vi "transferScanPatternToTarget.vi"(8 "error in (no error)":errorcluster, 10 "FPGA VI ref":T1, 11 "Queues":T2) -> (0 "error out":errorcluster)   [LabVIEW 2010]
uses:
  internal_queues.ctl
  line_info.ctl
  volume_with_lines.ctl
  volume_info.ctl
  kalman_result_scaled.ctl
  projection buffers.ctl
  location3D.ctl
  spot location.ctl
  FPGA_ref.ctl
  <vilib>/rvi/interface/nirviMethod/nirviMethod.xnode
  <vilib>/rvi/interface/common/niFpgaNodeNameForErrorReporting.ctl
  <vilib>/rvi/errors/niLvFpgaWhatHappensToTopLevelVI.ctl
  <vilib>/Utility/error.llb/Error Cluster From Error Code.vi
  <vilib>/rvi/errors/niLvFpgaAdjustHostInterfaceError.vi
  NiFpgaLv.dll
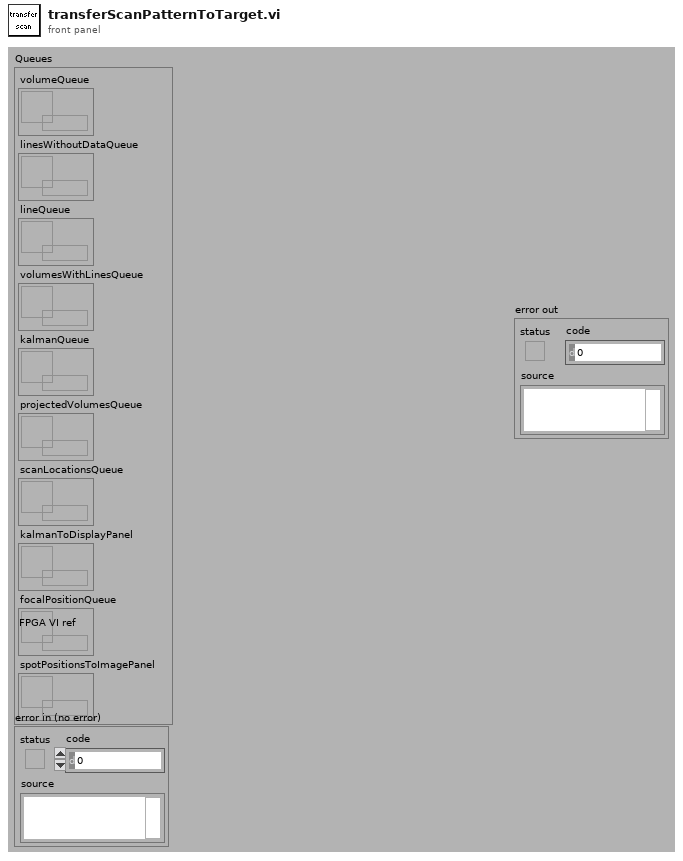
[diagram p1: front panel]
types:
  T1 = typedef "FPGA_ref.ctl" = refnum<k20>
  T2 = typedef "internal_queues.ctl" = cluster{"volumeQueue":refnum<queue>, "linesWithoutDataQueue":refnum<queue>, "lineQueue":refnum<queue>, "volumesWithLinesQueue":refnum<queue>, "kalmanQueue":refnum<queue>, "projectedVolumesQueue":refnum<queue>, "scanLocationsQueue":refnum<queue>, "kalmanToDisplayPanel":refnum<queue>, "focalPositionQueue":refnum<queue>, "spotPositionsToImagePanel":refnum<queue>}
  T3 = typedef "niFpgaNodeNameForErrorReporting.ctl" = enum16{"Open FPGA VI Reference", "Read/Write Control", "Invoke Method: Abort", "Invoke Method: Acknowledge IRQ", "Invoke Method: Download", "Invoke Method: FIFO.Configure", "Invoke Method: FIFO.Read", "Invoke Method: FIFO.Start", "Invoke Method: FIFO.Stop", "Invoke Method: FIFO.Write", "Invoke Method: Reset", "Invoke Method: Run", "Invoke Method: Wait on IRQ", "Close FPGA VI Reference"}
  T4 = typedef "niLvFpgaWhatHappensToTopLevelVI.ctl" = enum16{"top level VI scripted behind XNode", "top level VI inlined behind XNode"}
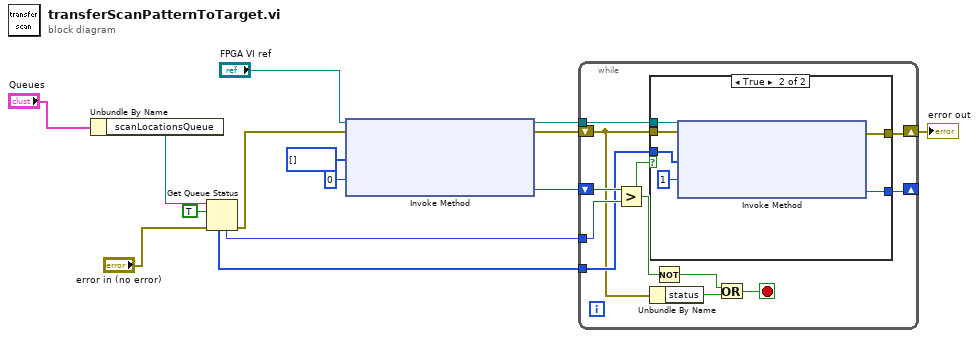
[diagram p0: block diagram]
diagram:
  n1 = Unbundle By Name("Queues") -> ("scanLocationsQueue"=w9:refnum<queue>)
  n2 = Get Queue Status(queue=w9, return elements? (F)=TRUE, error in (no error)="error in (no error)") -> (error out=w7:errorcluster, # elements in queue=w6:i32, elements=w5:u32[])  [unwired: 5 out]
  n3 = xnode "Invoke Method"("FPGA VI Reference In"="FPGA VI ref", "error in"=w7, "Data"=u32[] [], "Timeout (ms)"=0) -> ("FPGA VI Reference Out"=w2:T1, "error out"=w3:errorcluster, "Empty Elements Remaining"=w10:u32)
  n4 = while {
    shift-right: [w20] -> _
    shift-left: w10 -> [w25]
    tunnel: w6 -> [w24]
    tunnel: w5 -> [w21]
    tunnel: w2 -> [w22]
    shift-right: [w23] -> w1
    shift-left: w3 -> [w19]
    stop <- w15 stop-if-true
    n5 = Greater?(x=w25, y=w24) -> (0:w17:bool)
    n6 = case shown="True" w17 {
      tunnel: w19 -> [w26 w32]
      tunnel: [w26 w31] -> w23
      tunnel: w22 -> [_ w30]
      tunnel: w21 -> [_ w28]
      tunnel: [_ w27] -> w20
      frame False {
      }
      frame True {
        n7 = xnode "Invoke Method"("FPGA VI Reference In"=w30, "error in"=w32, "Data"=w28, "Timeout (ms)"=1) -> ("error out"=w31:errorcluster, "Empty Elements Remaining"=w27:u32)  [unwired: 1 out]
      }
    }
    n8 = Unbundle By Name(w19) -> ("status"=w18:bool)
    n9 = Not(x=w17) -> (.not. x?=w16:bool)
    n10 = Or(x=w16, y=w18) -> (x .or. y?=w15:bool)
  }
  "error out" <- w1
